vi "Get Port Status_UI Actor.vi"(8 "error in (no error)":errorcluster, 11 "UI Actor in":refnum<class "UI Actor.lvclass">) -> (0 "error out":errorcluster, 3 "UI Actor out":refnum<class "UI Actor.lvclass">)   [LabVIEW 2020, in "UI Actor.lvlib" / "UI Actor.lvclass"]
uses:
  UI Actor.lvclass
  UI Actor.lvclass/UI Actor.ctl
  Abstract/Serial Device/Serial Device.lvclass
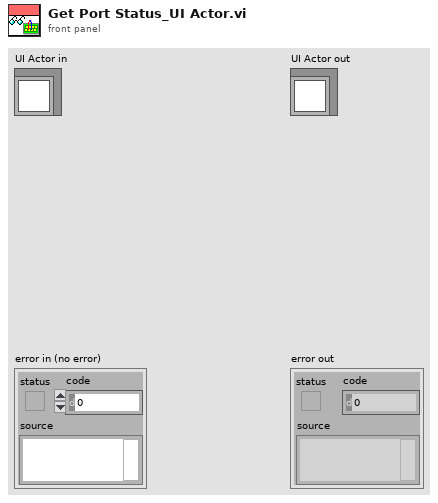
[diagram p1: front panel]
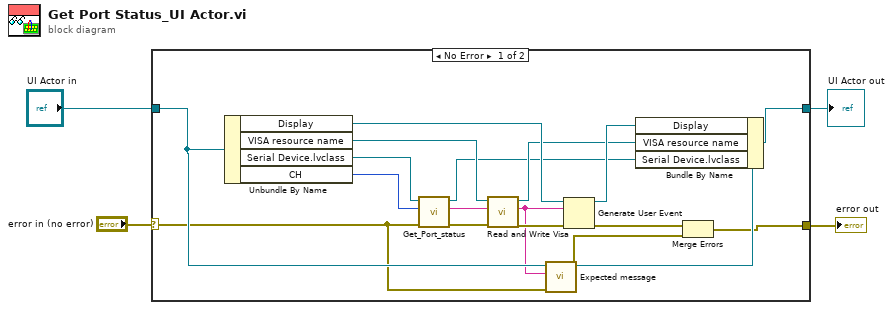
[diagram p0: block diagram]
diagram:
  n1 = case shown="No Error" "error in (no error)" {
    selector: "error in (no error)" -> [w5 w24]
    tunnel: [w7 w24] -> w3
    tunnel: [w16 w23] -> w1
    tunnel: "UI Actor in" -> [w11 w23]
    frame No Error {
      n2 = Unbundle By Name(w11) -> ("Display"=w22:refnum<user-event>, "VISA resource name"=w21:refnum<visa-resource-name>, "Serial Device.lvclass"=w17:refnum<class "Serial Device.lvclass">, "CH"=w12:i32)
      n3 = call-dynamic "Get_Port_status.vi"("error in (no error)"=w5, "CH"=w12, "Serial Device in"=w17) -> ("error out"=w14:errorcluster, "Command to Send"=w13:string, "Serial Device out"=w15:refnum<class "Serial Device.lvclass">)  [unwired: 5 in, 1 out]
      n4 = call "Read and Write Visa.vi"("error in (no error)"=w14, "Command to Send"=w13, "VISA Refnum in"=w21) -> ("error out"=w20:errorcluster, "Expected Response out"=w9:string, "VISA Refnum out"=w18:refnum<visa-resource-name>)  [unwired: 6 in]
      n5 = call "Expected message.vi"("error in (no error)"=w5, "Expected Response out"=w9, "UI Actor in"=w11) -> ("error IO"=w6:errorcluster, "UI Actor out"=w10:refnum<class "UI Actor.lvclass">)  [unwired: 7 in]
      n6 = Generate User Event(user event=w22, event data cluster=w9, error in=w20) -> (user event out=w19:refnum<user-event>, error out=w8:errorcluster)  [unwired: 1 in]
      n7 = Bundle By Name(cluster=w10, "Display"=w19, "VISA resource name"=w18, "Serial Device.lvclass"=w15) -> (w16:refnum<class "UI Actor.lvclass">)
      n8 = Merge Errors(w8, w6) -> (w7:errorcluster)
    }
    frame Error {
    }
  }
  "error out" <- w3
  "UI Actor out" <- w1
